vi "PXI-Flush Signal Bank.vi"(8 "error in (no error)":errorcluster) -> (0 "error out":errorcluster)   [LabVIEW 2020]
uses:
  DAQ Engine VIs/PXI Globals.vi
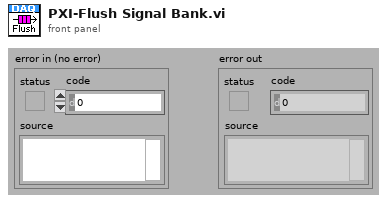
[diagram p1: front panel]
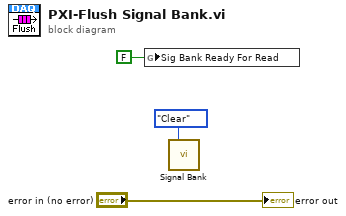
[diagram p0: block diagram]
diagram:
  n1 = global write "PXI Globals.vi" "Sig Bank Ready For Read"(FALSE ("Sig Bank Ready For Read")) -> ()
  n2 = call "Signal Bank.vi"("Action"=enum16{"Add", "Replace ID", "Read ID", "Clear"}."Clear") -> ()  [unwired: 13 in, 2 out]
  "error out" <- "error in (no error)"
